vi "Result_Test.vi"(8 "error in (no error)":errorcluster caption="entrée d'erreur (pas d'erreur)", 11 "Flash_Jlink en entrée":refnum<class "Check_State.lvclass">) -> (0 "error out":errorcluster caption="sortie d'erreur", 3 "Flash_Jlink en sortie":refnum<class "Check_State.lvclass">)   [LabVIEW 2020, in "Library Test.lvlib" / "Check_State.lvclass"]
uses:
  Check_State.lvclass
  C:/Users/ngarcin/OneDrive - Altyor/Standard TB/Suite TB45/Class/Test/Test (Default)/Test (Default).lvclass
  Commun VI/TypeDef/Variable Printable.ctl
  Test_Without_Instr/Test_Without_Inst.lvclass
  Commun VI/Library Commun.lvlib
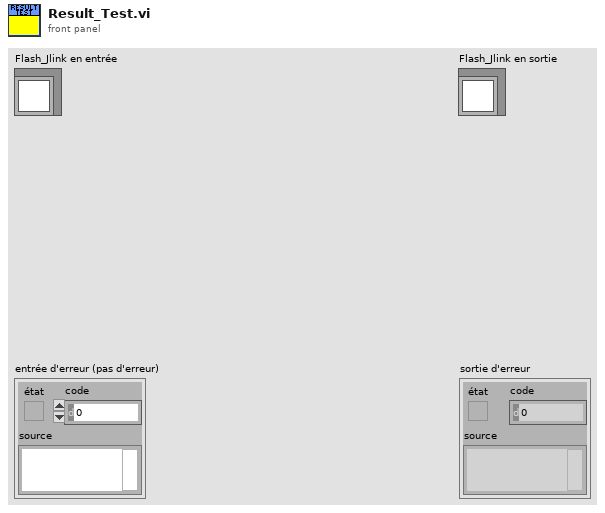
[diagram p1: front panel]
types:
  T1 = enum16{"Get Variable", "Get All Variables", "Set Variable", "Delete Variable", "Delete All Variable"}
  T2 = typedef "Variable Printable.ctl" = string
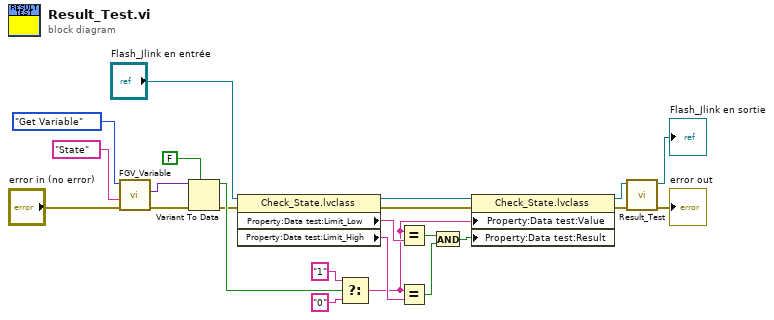
[diagram p0: block diagram]
diagram:
  n1 = call "FGV_Variable.vi"("error in (no error)"="error in (no error)", "Variable"=T2 "State", "Function"=T1."Get Variable") -> ("error out"=w17:errorcluster, "Data Out"=w16:variant)  [unwired: 6 in, 1 out]
  n2 = Variant To Data(error in=w17, type=FALSE, Variant=w16) -> (data=w13:bool, error out=w4:errorcluster)
  n3 = property class="Check_State.lvclass"(reference="Flash_Jlink en entrée", error in=w4) -> (reference out=w3:refnum<class "Check_State.lvclass">, error out=w2:errorcluster, "Property:Data test:Limit_Low"=w9:string, "Property:Data test:Limit_High"=w8:string)
  n4 = Select(t="1" ("y"), s=w13, f="0" ("y")) -> (s? t:f=w1:string)
  n5 = Equal?(x=w1, y=w9) -> (x = y?=w7:bool)
  n6 = Equal?(x=w1, y=w8) -> (x = y?=w6:bool)
  n7 = And(x=w7, y=w6) -> (x .and. y?=w5:bool)
  n8 = property class="Check_State.lvclass"(reference=w3, error in=w2, "Property:Data test:Value"=w1, "Property:Data test:Result"=w5) -> (reference out=w20:refnum<class "Check_State.lvclass">, error out=w21:errorcluster)
  n9 = call-parent "Result_Test.vi"("error in (no error)"=w21, "Test_Without_Inst en entrée"=w20) -> ("error out"=→"error out":errorcluster, "Test_Without_Inst en sortie"=→"Flash_Jlink en sortie":refnum<class "Check_State.lvclass">)  [unwired: 8 in]
